vi "DC Power.vi"() -> ()   [LabVIEW 2023]
panel:
  in  "VISA resource name 4":refnum<visa-resource-name>
  in  "VISA resource name 2":refnum<visa-resource-name>
  in  "VISA resource name 3":refnum<visa-resource-name>
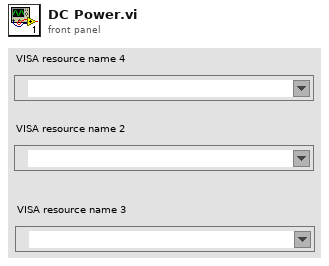
[diagram p1: front panel]
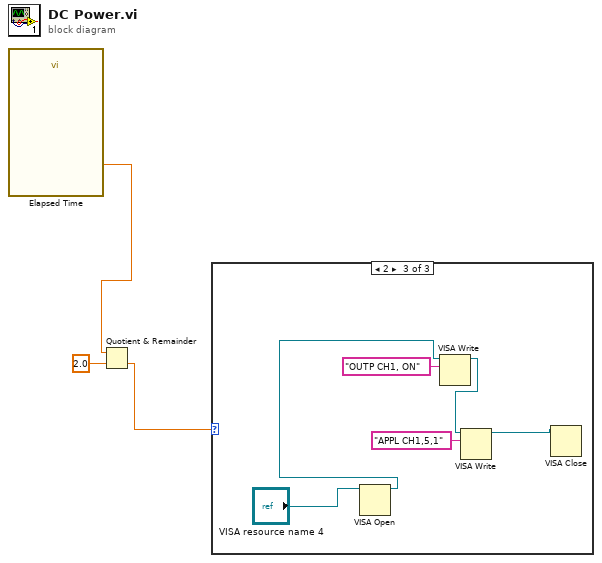
[diagram p0: block diagram]
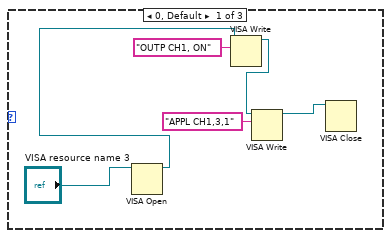
[diagram p2: hidden frame]
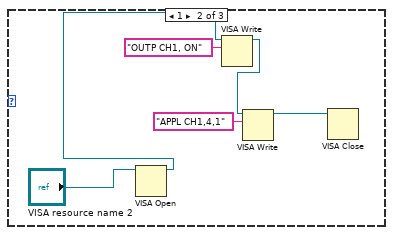
[diagram p3: hidden frame]
diagram:
  n1 = call "Elapsed Time"() -> ("Elapsed Time (s)"=w1:dbl)  [unwired: 12 in, 7 out]
  n2 = Quotient & Remainder(x=w1, y=2.0) -> (floor(x/y)=w2:dbl)  [unwired: 1 out]
  n3 = case shown="2" w2 {
    frame 0, Default {
      n4 = VISA Open(VISA resource name="VISA resource name 3") -> (VISA resource name=w5:refnum<visa-resource-name>)  [unwired: 4 in, 1 out]
      n5 = VISA Write(VISA resource name=w5, write buffer="OUTP CH1, ON") -> (VISA resource name out=w8:refnum<visa-resource-name>)  [unwired: 1 in, 2 out]
      n6 = VISA Write(VISA resource name=w8, write buffer="APPL CH1,3,1") -> (VISA resource name out=w4:refnum<visa-resource-name>)  [unwired: 1 in, 2 out]
      n7 = VISA Close(VISA resource name=w4) -> ()  [unwired: 1 in, 1 out]
    }
    frame 1 {
      n8 = VISA Open(VISA resource name="VISA resource name 2") -> (VISA resource name=w11:refnum<visa-resource-name>)  [unwired: 4 in, 1 out]
      n9 = VISA Write(VISA resource name=w11, write buffer="OUTP CH1, ON") -> (VISA resource name out=w14:refnum<visa-resource-name>)  [unwired: 1 in, 2 out]
      n10 = VISA Write(VISA resource name=w14, write buffer="APPL CH1,4,1") -> (VISA resource name out=w10:refnum<visa-resource-name>)  [unwired: 1 in, 2 out]
      n11 = VISA Close(VISA resource name=w10) -> ()  [unwired: 1 in, 1 out]
    }
    frame 2 {
      n12 = VISA Open(VISA resource name="VISA resource name 4") -> (VISA resource name=w17:refnum<visa-resource-name>)  [unwired: 4 in, 1 out]
      n13 = VISA Write(VISA resource name=w17, write buffer="OUTP CH1, ON") -> (VISA resource name out=w20:refnum<visa-resource-name>)  [unwired: 1 in, 2 out]
      n14 = VISA Write(VISA resource name=w20, write buffer="APPL CH1,5,1") -> (VISA resource name out=w16:refnum<visa-resource-name>)  [unwired: 1 in, 2 out]
      n15 = VISA Close(VISA resource name=w16) -> ()  [unwired: 1 in, 1 out]
    }
  }
